vi "Check Status.vi"(8 "error in (no error)":errorcluster, 11 "Power Supply in":refnum<class "Power Supply.lvclass">) -> (0 "error out":errorcluster, 1 "Status":string, 2 "Ready?":bool, 3 "Power Supply out":refnum<class "Power Supply.lvclass">)   [LabVIEW 2009, in "Power Supply.lvclass"]
uses:
  Power Supply.lvclass
  Power Supply.lvclass/Power Supply.ctl
panel:
  out "switchheater":bool caption="Switch Heater"
  out "persis?":bool caption="Persistent Mode"
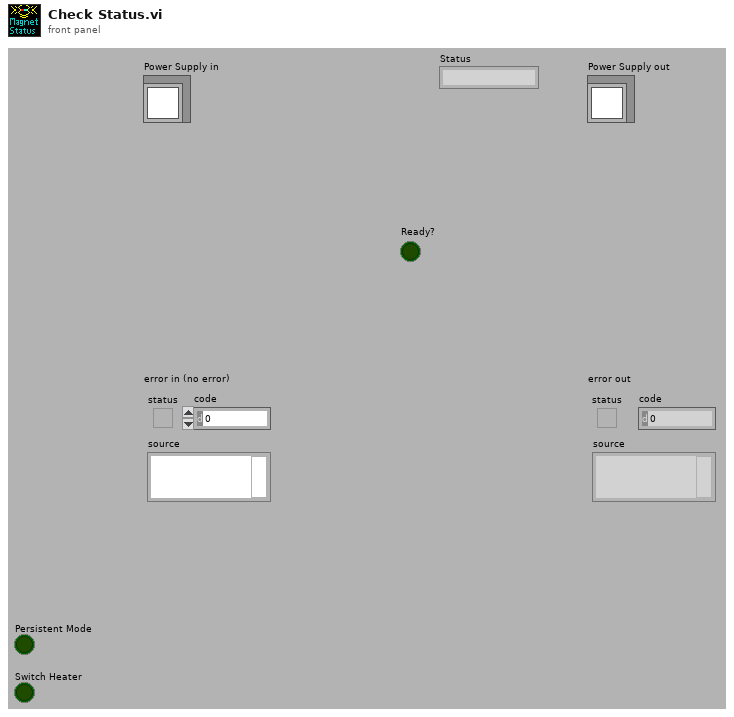
[diagram p1: front panel]
types:
  T1 = typedef "OxfordAddress.ctl" = cluster{"Com Port":i32, "ISOBUS Address":i32, "GPIB Address":i16, "Communication":enum16{"RS232", "ISOBUS", "GPIB", "Gateway"}}
  T2 = typedef "PSIO.ctl" = cluster{"Address":T1, "Version":enum16{"PS", "IPS"}}
  T3 = cluster{"Value":i16, "At rest":bool, "Sweeping":bool, "Rate limiting":bool}
  T4 = cluster{"Value":i16, "Hold":bool, "To set point":bool, "To zero":bool, "Clamped":bool}
  T5 = cluster{"Value":i16, "Off (at zero field)":bool, "On":bool, "Off (at field)":bool, "No switch fitted":bool, "Confirm":bool}
  T6 = cluster{"Value":i16, "Quenched":bool, "Over heated":bool, "Warming up":bool}
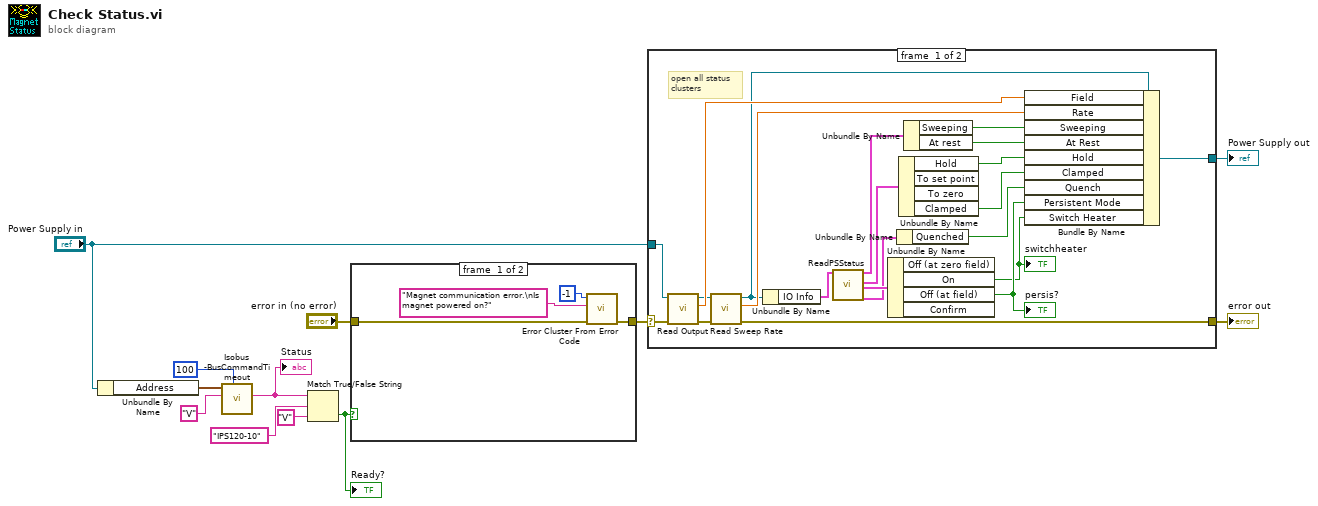
[diagram p0: block diagram]
diagram:
  n1 = Unbundle By Name("Power Supply in") -> ("Address"=w6:T1)
  n2 = call "Isobus -BusCommandTimeout.vi"("Timeout (ms)"=100, "Command"="V", "Address"=w6) -> ("Reply"=w10:string)  [unwired: 5 out]
  "Status" <- w10
  n3 = Match True/False String(2:"V", 3:"IPS120-10", 4:w10) -> (0:w1:bool)  [unwired: 1 out]
  "Ready?" <- w1
  n4 = case shown="False" w1 {
    tunnel: "error in (no error)" -> [w14 w17]
    tunnel: [w13 w17] -> w2
    frame #0 {
      n5 = call <vilib>:"Error Cluster From Error Code.vi"("error in (no error)"=w14, "error message (\"\")"="Magnet communication error.\nIs magnet powered on?" ("error message (\"\")"), "error code (0)"=-1) -> ("error out"=w13:errorcluster)  [unwired: 6 in]
    }
    frame #1 {
    }
  }
  n6 = case shown="No Error" w2 {
    selector: w2 -> [w21 w39]
    tunnel: "Power Supply in" -> [w24 w40]
    tunnel: [w25 w40] -> w12
    tunnel: [w20 w39] -> w11
    frame #0 {
      # "open all status\nclusters"
      n7 = call-dynamic "Read Output.vi"("error in (no error)"=w21, "Power Supply in"=w24) -> ("error out"=w22:errorcluster, "Field"=w27:dbl[unit], "Power Supply out"=w23:refnum<class "Power Supply.lvclass">)  [unwired: 6 in, 1 out]
      n8 = call-dynamic "Read Sweep Rate.vi"("error in (no error)"=w22, "Power Supply in"=w23) -> ("error out"=w20:errorcluster, "Field sweep rate"=w26:dbl[unit], "Power Supply out"=w19:refnum<class "Power Supply.lvclass">)  [unwired: 7 in]
      n9 = Unbundle By Name(w19) -> ("IO Info"=w18:T2)
      n10 = call "ReadPSStatus.vi"("IO Info"=w18) -> ("Mode (n)"=w36:T3, "Activity"=w38:T4, "Switch Heater"=w37:T5, "System Status (m)"=w35:T6)  [unwired: 15 out]
      n11 = Unbundle By Name(w37) -> ("On"=w28:bool, "Off (at field)"=w29:bool)  [unwired: 2 out]
      "persis?" <- w29
      "switchheater" <- w28
      n12 = Unbundle By Name(w35) -> ("Quenched"=w32:bool)
      n13 = Unbundle By Name(w38) -> ("Hold"=w30:bool, "Clamped"=w33:bool)  [unwired: 2 out]
      n14 = Unbundle By Name(w36) -> ("Sweeping"=w34:bool, "At rest"=w31:bool)
      n15 = Bundle By Name(cluster=w19, "Field"=w27, "Rate"=w26, "Sweeping"=w34, "At Rest"=w31, "Hold"=w30, "Clamped"=w33, "Quench"=w32, "Persistent Mode"=w29, "Switch Heater"=w28) -> (w25:refnum<class "Power Supply.lvclass">)
    }
    frame #1 {
    }
  }
  "Power Supply out" <- w12
  "error out" <- w11
